vi "NicmosOpenSynchronization.vi"(9 "error out":errorcluster caption="error in (no error)") -> (2 "Synchronization":T1, 6 "error in (no error)":errorcluster caption="error out")   [LabVIEW 2009]
uses:
  Controls/NicmosSynchronization.ctl
  Controls/NICMOS.COMMAND.ctl
  Controls/NICMOS.COMMANDBASIC.ctl
  Controls/NICMOS.READOUT.ctl
  Controls/NICMOS.FILTERCOMMAND.ctl
  Controls/NICMOS.FILTER.ctl
  Controls/NICMOS.STATE.ctl
  Controls/NICMOS.DATA.ctl
  Controls/NICMOS.RAW.ctl
  Controls/NICMOS.TEMPERATURE.ctl
  Controls/NICMOS.MASKBANKS.ctl
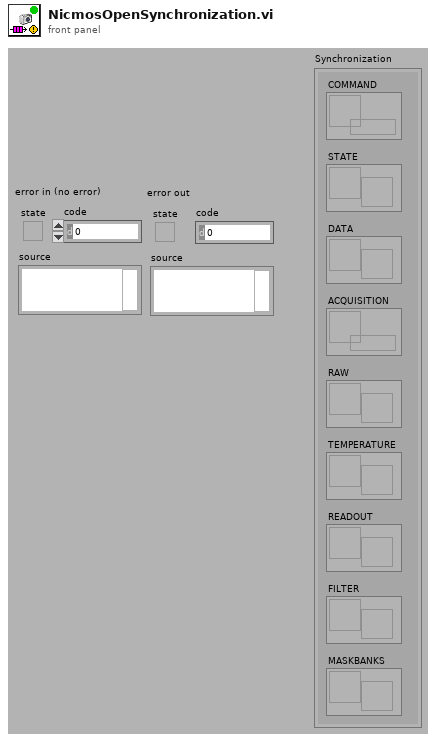
[diagram p1: front panel]
types:
  T1 = typedef "NicmosSynchronization.ctl" = cluster{"COMMAND":refnum<queue>, "STATE":refnum<notifier>, "DATA":refnum<notifier>, "ACQUISITION":refnum<queue>, "RAW":refnum<notifier>, "TEMPERATURE":refnum<notifier>, "READOUT":refnum<notifier>, "FILTER":refnum<notifier>, "MASKBANKS":refnum<notifier>}
  T2 = typedef "NICMOS.MASKBANKS.ctl" = cluster{"MaskList":cluster{"X":i32, "Y":i32, "NX":i32, "NY":i32}[], "Reform X":i32, "Reform Y":i32}[]
  T3 = typedef "NICMOS.FILTER.ctl" = string
  T4 = typedef "NICMOS.READOUT.ctl" = cluster{"Readout":i32, "Deglitch":i32, "Framerate":dbl[unit], "Bank":i32}
  T5 = typedef "NICMOS.TEMPERATURE.ctl" = cluster{"T1":dbl, "T2":dbl}
  T6 = typedef "NICMOS.DATA.ctl" = cluster{"DATA":i32[][][], "INDEX":i32}
  T7 = typedef "NICMOS.COMMAND.ctl" = cluster{"Command":T8, "READOUT":T4, "FILTERCOMMAND":T9, "ACQUISITION":i32, "Done":refnum<k4>}
  T8 = typedef "NICMOS.COMMANDBASIC.ctl" = enum16{"WRITE BANKS", "SET FILTER", "HOME FILTER", "QUERY TEMP", "CONFIGURE", "START", "ACQUISITION", "STOP", "QUIT"}
  T9 = typedef "NICMOS.FILTERCOMMAND.ctl" = cluster{"FILTER":T3, "INIT":bool}
  T10 = typedef "NICMOS.STATE.ctl" = enum16{"IDLE", "WRITING BANKS", "SETTING FILTER", "HOMING FILTER", "QUERYING TEMP", "CONFIGURING", "STARTING", "RUNNING", "HALTING", "STOPPED"}
  T11 = typedef "NICMOS.RAW.ctl" = u16[][][]
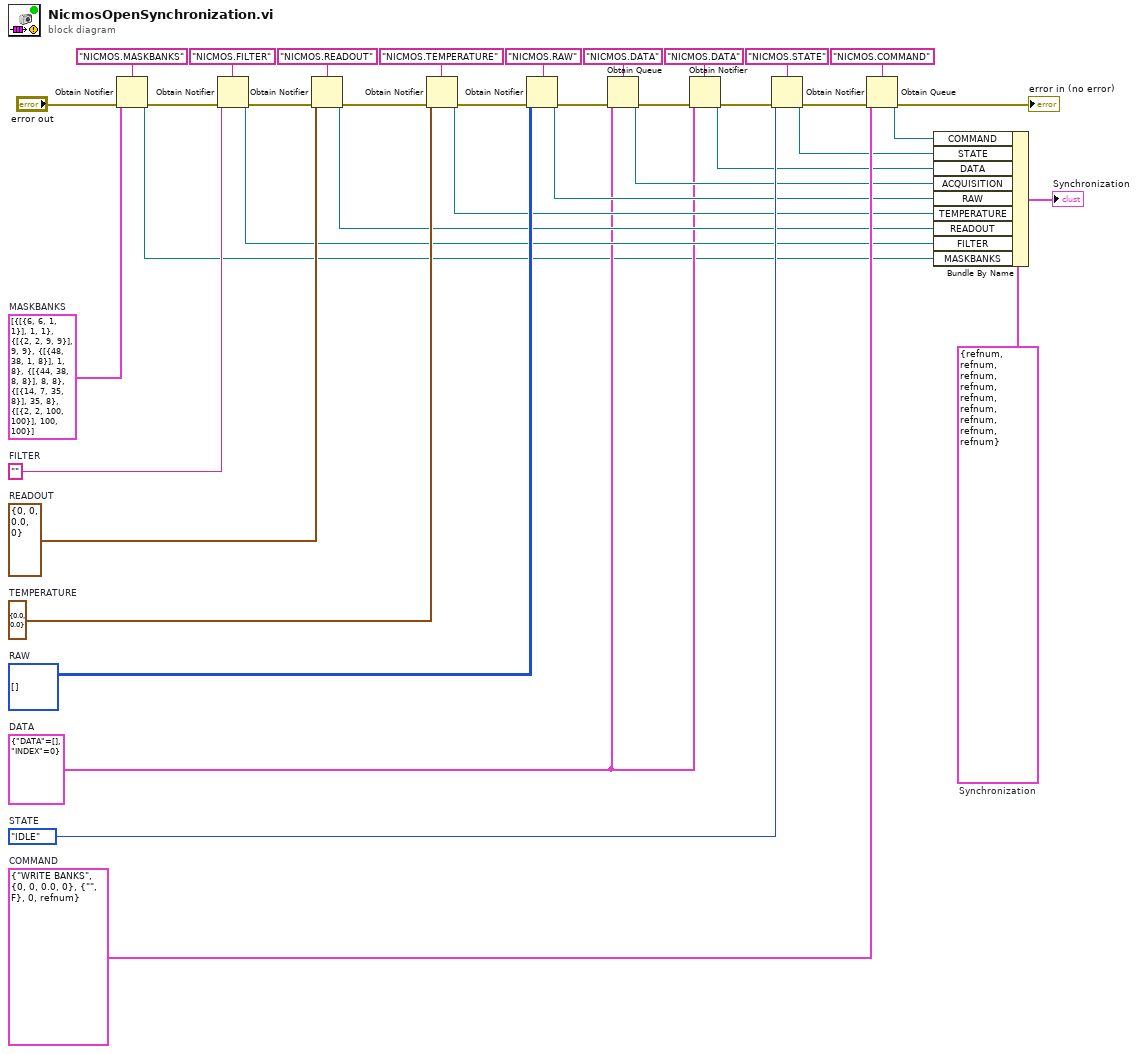
[diagram p0: block diagram]
diagram:
  w1 = T1 {"COMMAND"=refnum, "STATE"=refnum, "DATA"=refnum, "ACQUISITION"=refnum, "RAW"=refnum, "TEMPERATURE"=refnum, "READOUT"=refnum, "FILTER"=refnum, "MASKBANKS"=refnum}  # Synchronization
  w5 = T2 [{"MaskList"=[{"X"=6, "Y"=6, "NX"=1, "NY"=1}], "Reform X"=1, "Reform Y"=1}, {"MaskList"=[{"X"=2, "Y"=2, "NX"=9, "NY"=9}], "Reform X"=9, "Reform Y"=9}, {"MaskList"=[{"X"=48, "Y"=38, "NX"=1, "NY"=8}], "Reform X"=1, "Reform Y"=8}, {"MaskList"=[{"X"=44, "Y"=38, "NX"=8, "NY"=8}], "Reform X"=8, "Reform Y"=8}, {"MaskList"=[{"X"=14, "Y"=7, "NX"=35, "NY"=8}], "Reform X"=35, "Reform Y"=8}, {"MaskList"=[{"X"=2, "Y"=2, "NX"=100, "NY"=100}], "Reform X"=100, "Reform Y"=100}]  # MASKBANKS
  w15 = T3 ""  # FILTER
  w18 = T4 {"Readout"=0, "Deglitch"=0, "Framerate"=0.0, "Bank"=0}  # READOUT
  w21 = T5 {"T1"=0.0, "T2"=0.0}  # TEMPERATURE
  w9 = T6 {"DATA"=[], "INDEX"=0}  # DATA
  w29 = T7 {"Command"=enum."WRITE BANKS", "READOUT"={"Readout"=0, "Deglitch"=0, "Framerate"=0.0, "Bank"=0}, "FILTERCOMMAND"={"FILTER"="", "INIT"=FALSE}, "ACQUISITION"=0, "Done"=refnum}  # COMMAND
  w31 = NICMOS.STATE."IDLE"  # STATE
  w30 = T11 []  # RAW
  n1 = Obtain Notifier(name (unnamed)="NICMOS.MASKBANKS" ("nom (aucun)"), notification data type=w5, error in (no error)="error out") -> (notifier out=w4:refnum<notifier>, error out=w6:errorcluster)  [unwired: 1 in, 1 out]
  n2 = Obtain Notifier(name (unnamed)="NICMOS.FILTER" ("nom (aucun)"), notification data type=w15, error in (no error)=w6) -> (notifier out=w14:refnum<notifier>, error out=w3:errorcluster)  [unwired: 1 in, 1 out]
  n3 = Obtain Notifier(name (unnamed)="NICMOS.READOUT" ("nom (aucun)"), notification data type=w18, error in (no error)=w3) -> (notifier out=w17:refnum<notifier>, error out=w2:errorcluster)  [unwired: 1 in, 1 out]
  n4 = Obtain Notifier(name (unnamed)="NICMOS.TEMPERATURE" ("nom (aucun)"), notification data type=w21, error in (no error)=w2) -> (notifier out=w20:refnum<notifier>, error out=w22:errorcluster)  [unwired: 1 in, 1 out]
  n5 = Obtain Notifier(name (unnamed)="NICMOS.RAW" ("nom (aucun)"), notification data type=w30, error in (no error)=w22) -> (notifier out=w24:refnum<notifier>, error out=w32:errorcluster)  [unwired: 1 in, 1 out]
  n6 = Obtain Queue(name (unnamed)="NICMOS.DATA" ("nom (aucun)"), element data type=w9, error in (no error)=w32) -> (queue out=w25:refnum<queue>, error out=w13:errorcluster)  [unwired: 2 in, 1 out]
  n7 = Obtain Notifier(name (unnamed)="NICMOS.DATA" ("nom (aucun)"), notification data type=w9, error in (no error)=w13) -> (notifier out=w10:refnum<notifier>, error out=w12:errorcluster)  [unwired: 1 in, 1 out]
  n8 = Obtain Notifier(name (unnamed)="NICMOS.STATE" ("nom (aucun)"), notification data type=w31, error in (no error)=w12) -> (notifier out=w26:refnum<notifier>, error out=w34:errorcluster)  [unwired: 1 in, 1 out]
  n9 = Obtain Queue(name (unnamed)="NICMOS.COMMAND" ("nom (aucun)"), element data type=w29, error in (no error)=w34) -> (queue out=w27:refnum<queue>, error out=→"error in (no error)":errorcluster)  [unwired: 2 in, 1 out]
  n10 = Bundle By Name(cluster=w1, "COMMAND"=w27, "STATE"=w26, "DATA"=w10, "ACQUISITION"=w25, "RAW"=w24, "TEMPERATURE"=w20, "READOUT"=w17, "FILTER"=w14, "MASKBANKS"=w4) -> (→"Synchronization":T1)
